vi "SaveCheck.vi"(8 "error in (no error)":errorcluster, 10 "DataTable In":string[][](array[string]), 11 "Data In":T1) -> (0 "error out":errorcluster, 1 "Save Data":string[](array[string]), 2 "DataTable Out":string[][](array[string]), 3 "Data Out":T1, 4 "IT Save?":bool, 5 "Dupicate":bool, 6 "index (row)":i32=7)   [LabVIEW 2014]
uses:
  controls/Data1.ctl
  controls/Payjson.ctl
panel:
  out "CarNo":string
  out "OK?":bool
  out "CARNO":i32
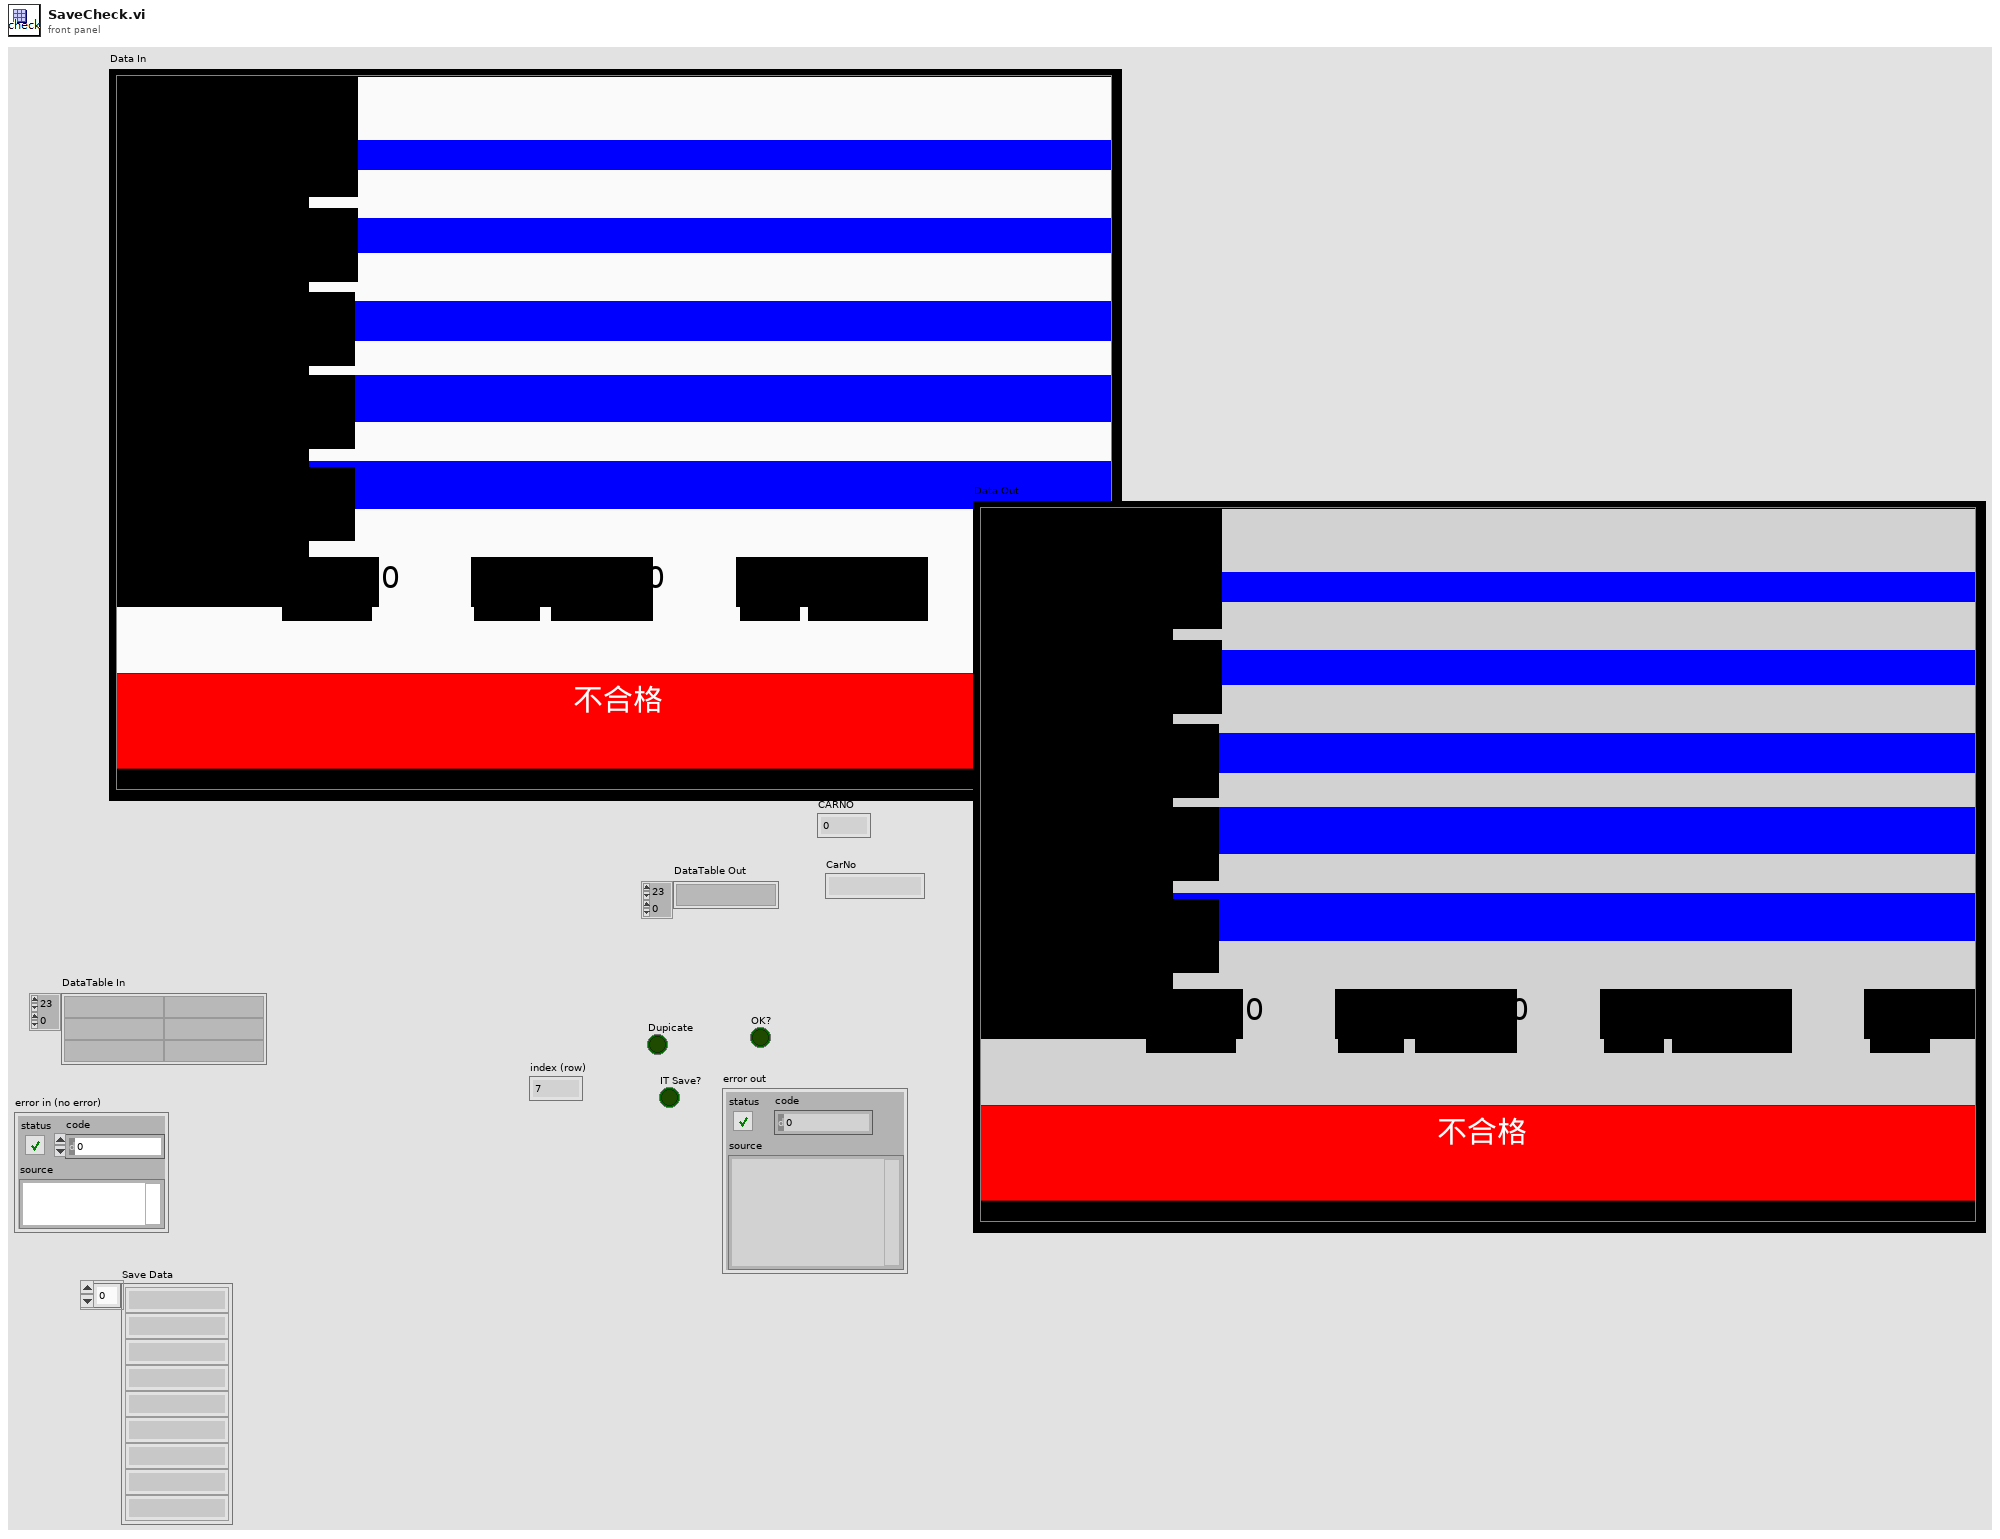
[diagram p1: front panel]
types:
  T1 = typedef "Data1.ctl" = cluster{"Date":string, "BarCode1":string, "BarCode2":string, "BarCode3":string, "Message":string, "OK Count":u16, "NG Count":u16, "Total Count":u16, "ModelData":string[][], "OK&NG":bool, "COM1":refnum<visa-resource-name>, "COM2":refnum<visa-resource-name>, "IO":i32, "Time":u32, "TCP":refnum<k5>, "TCP 2":refnum<k5>, "COM1 2":refnum<visa-resource-name>, "CheckNum":string, "BarCode1_1":string, "BarCode2_1":string, "BarCode3_1":string, "日期":string, "機種":string, "機號":string, "商品條碼1":string, "OK_1":string, "OK":string, "NG":string, "NG_1":string, "Total":string, "Total_1":string, "ClaerTime":u32, "Pjson":T2, "LotNo":string[], "CheckParsArray":string[], "BarCode4":string, "BarCode4_1":string, "商品條碼2":string, "BarCode5":string, "BarCode5_1":string, "商品條碼3":string, "ReScanNG":i32, "NGTimeCT":u32}
  T2 = typedef "Payjson.ctl" = cluster{"DEPT":string, "LINE":string, "STANO":string, "WORKNO":string, "PRODSN":string, "COMPNTID":string, "COMPNTLOT":string, "COMPNTSN":string, "USEDQTY":i16, "OPDATE":string, "OPUSER":string, "RECVDATE":string, "MMODU":string}[]
  T3 = cluster{"DEPT":string, "LINE":string, "STANO":string, "WORKNO":string, "PRODSN":string, "COMPNTID":string, "COMPNTLOT":string, "COMPNTSN":string, "USEDQTY":i16, "OPDATE":string, "OPUSER":string, "RECVDATE":string, "MMODU":string}
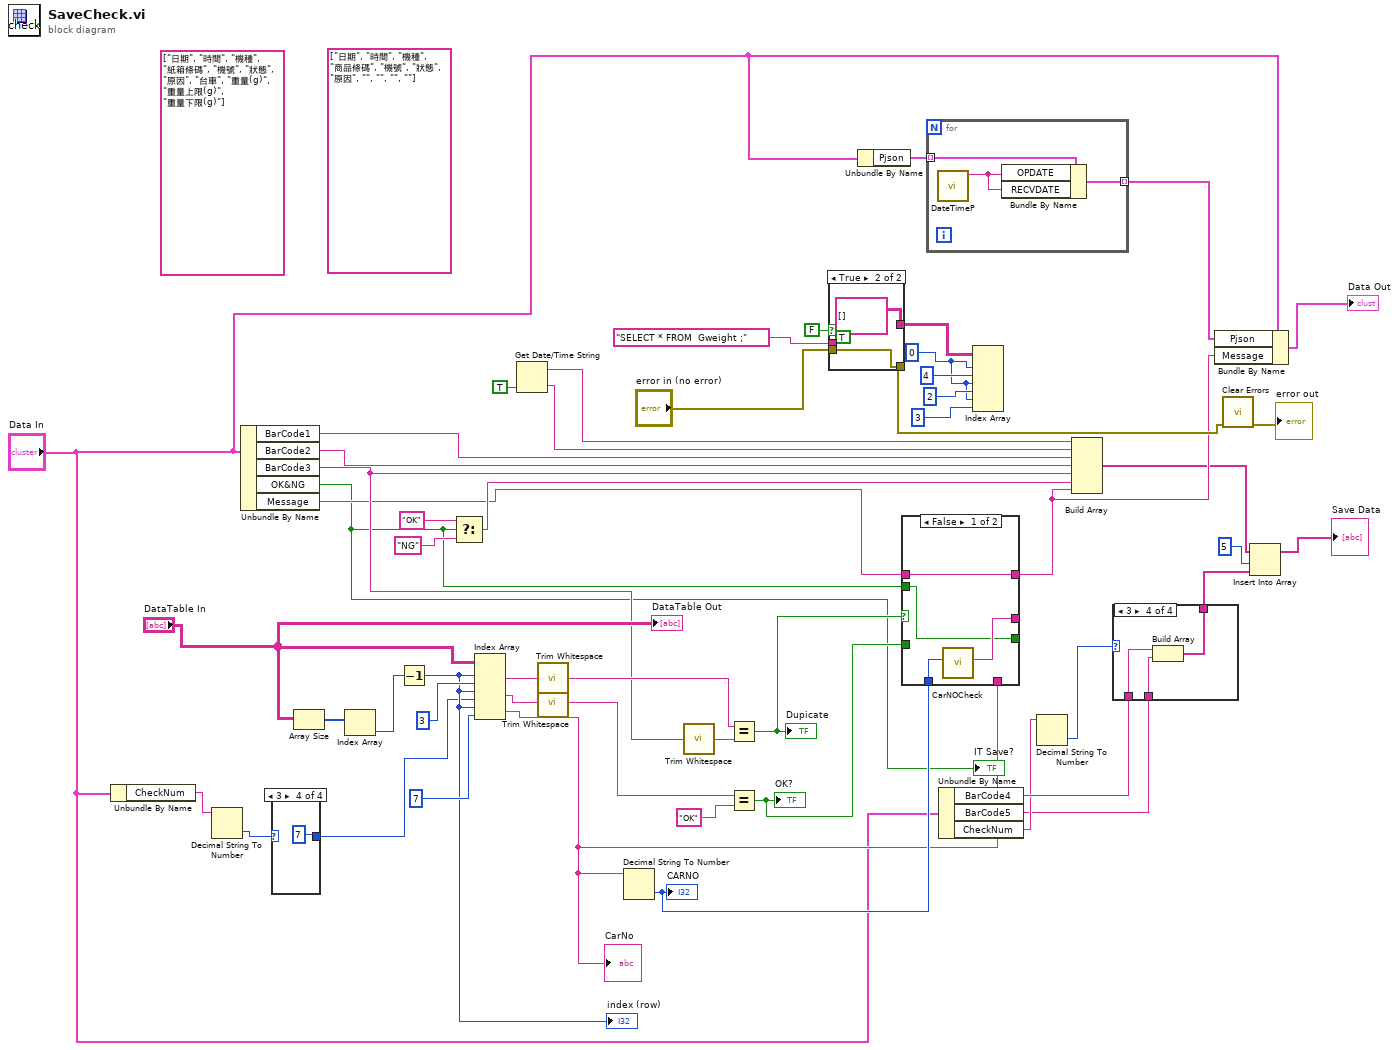
[diagram p0: block diagram]
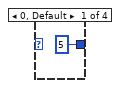
[diagram p2: hidden frame]
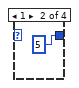
[diagram p3: hidden frame]
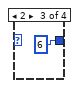
[diagram p4: hidden frame]
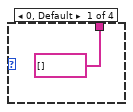
[diagram p5: hidden frame]
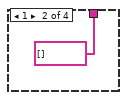
[diagram p6: hidden frame]
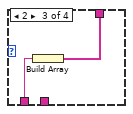
[diagram p7: hidden frame]
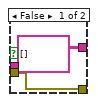
[diagram p8: hidden frame]
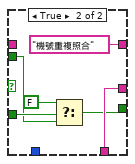
[diagram p9: hidden frame]
diagram:
  (unwired) string[] ["日期", "時間", "機種", "紙箱條碼", "機號", "狀態", "原因", "台車", "重量(g)", "重量上限(g)", "重量下限(g)"]
  w24 = 0 ("disabled index (row)")
  (unwired) string[] ["日期", "時間", "機種", "商品條碼", "機號", "狀態", "原因", "", "", "", ""]
  n1 = Unbundle By Name("Data In") -> ("CheckNum"=w5:string)
  n2 = Decimal String To Number(string=w5) -> (number=w4:i32)  [unwired: 2 in, 1 out]
  n3 = Unbundle By Name("Data In") -> ("BarCode1"=w40:string, "BarCode2"=w38:string, "BarCode3"=w19:string, "OK&NG"=w10:bool, "Message"=w18:string)
  "IT Save?" <- w10
  n4 = case shown="3" w4 {
    tunnel: [5 ("index (row)") 5 ("index (row)") 6 ("index (row)") 7 ("index (row)")] -> w3
    frame 0, Default {
    }
    frame 1 {
    }
    frame 2 {
    }
    frame 3 {
    }
  }
  n5 = Array Size(array="DataTable In") -> (size(s)=w53:i32[])
  n6 = Index Array(array=w53) -> (element=w45:i32)  [unwired: 1 in]
  n7 = Decrement(x=w45) -> (x-1=w44:i32)
  "index (row)" <- w44
  n8 = Select(t="OK", s=w10, f="NG") -> (s? t:f=w39:string)
  n9 = Index Array(array="DataTable In", index (row) #1=w44, index (col) #1=3 ("disabled index (col)"), index (row) #2=w44, index (col) #2=w3, index (row) #3=w44, index (col) #3=7 ("index (row)")) -> (element #1=w50:string, element #2=w48:string, element #3=w33:string)
  "CarNo" <- w33
  n10 = Get Date/Time String(want seconds? (F)=TRUE) -> (date string=w36:string, time string=w37:string)  [unwired: 2 in]
  n11 = call <vilib>:"Trim Whitespace.vi"("string"=w50) -> ("trimmed string"=w52:string)  [unwired: 1 in]
  n12 = call <vilib>:"Trim Whitespace.vi"("string"=w48) -> ("trimmed string"=w46:string)  [unwired: 1 in]
  n13 = Decimal String To Number(string=w33) -> (number=w34:i32)  [unwired: 2 in, 1 out]
  "CARNO" <- w34
  n14 = call <vilib>:"Trim Whitespace.vi"("string"=w19) -> ("trimmed string"=w43:string)  [unwired: 1 in]
  n15 = Equal?(x=w52, y=w43) -> (x = y?=w31:bool)
  "Dupicate" <- w31
  n16 = Equal?(x=w46, y="OK") -> (x = y?=w16:bool)
  "OK?" <- w16
  n17 = case shown="True" FALSE {
    tunnel: "SELECT * FROM  Gweight ;" ("CommandText") -> [_ _]
    tunnel: [string[][] [] ("Data") string[][] [] ("Data")] -> w29
    tunnel: "error in (no error)" -> [w59 w60]
    tunnel: [w59 w60] -> w22
    frame False {
    }
    frame True {
      (unwired) TRUE ("出資料")
    }
  }
  n18 = Unbundle By Name("Data In") -> ("Pjson"=w2:T2)
  n19 = case shown="False" w31 {
    tunnel: w34 -> [w65 _]
    tunnel: [w64 w71] -> _
    tunnel: w33 -> [_ w71]
    tunnel: w16 -> [_ w70]
    tunnel: w10 -> [w63 w69]
    tunnel: [w63 w67] -> _
    tunnel: w18 -> [w62 _]
    tunnel: [w62 "機號重複照合" ("Message")] -> w17
    frame False {
      n20 = call "CarNOCheck.vi"("CARNO"=w65) -> ("CarNO"=w64:string)  [unwired: 10 in]
    }
    frame True {
      n21 = Select(t=FALSE, s=w70, f=w69) -> (s? t:f=w67:bool)
    }
  }
  n22 = for {
    tunnel: w2 -> [w74] mode=indexing
    tunnel: [w72] -> w1 mode=indexing
    n23 = call "DateTimeP.vi"() -> ("date/time string"=w73:string)  [unwired: 11 in]
    n24 = Bundle By Name(cluster=w74, "OPDATE"=w73, "RECVDATE"=w73) -> (w72:T3)
  }
  n25 = Unbundle By Name("Data In") -> ("BarCode4"=w9:string, "BarCode5"=w7:string, "CheckNum"=w8:string)
  n26 = Index Array(array=w29, index (row) #1=w24, index (col) #1=4 ("disabled index (col)"), index (row) #2=w24, index (col) #2=2 ("disabled index (col)"), index (row) #3=w24, index (col) #3=3 ("disabled index (col)")) -> ()  [unwired: 3 out]
  n27 = Decimal String To Number(string=w8) -> (number=w12:i32)  [unwired: 2 in, 1 out]
  n28 = Build Array(w36, w37, w40, w38, w19, w39, w17) -> (w15:string[])
  n29 = case shown="3" w12 {
    tunnel: [string[] [] string[] [] w77 w79] -> w11
    tunnel: w9 -> [_ _ w78 w81]
    tunnel: w7 -> [_ _ _ w80]
    frame 0, Default {
    }
    frame 1 {
    }
    frame 2 {
      n30 = Build Array(w78) -> (w77:string[])
    }
    frame 3 {
      n31 = Build Array(w81, w80) -> (w79:string[])
    }
  }
  n32 = Bundle By Name(cluster="Data In", "Pjson"=w1, "Message"=w17) -> (→"Data Out":T1)
  n33 = call <vilib>:"Clear Errors.vi"("error in (no error)"=w22) -> ("error out"=→"error out":errorcluster)  [unwired: 5 in, 1 out]
  n34 = Insert Into Array(array=w15, index=5, new element=w11) -> (→"Save Data":string[])
  "DataTable Out" <- "DataTable In"
